vi "ALTS-2015 Prev Test Result Read DB Driver.vi"(7 "Cases":T1, 8 "error in (no error)":errorcluster, 11 "Serial Number":string) -> (0 "error out":errorcluster, 1 "Prev AirLeak result":string, 2 "Non-Empty Data from DB?":bool, 3 "data":string[][](array[string]))   [LabVIEW 2013]
doc: "Copyright © 2005, Soliton Technologies.\nAll rights reserved."
uses:
  <vilib>/addons/database/Auxilliary.llb/DB Tools Parameter Info.ctl
  <vilib>/addons/database/Auxilliary.llb/DB Tools DataTypes.ctl
  <vilib>/addons/database/Auxilliary.llb/DB Tools Parameter Dir.ctl
  Controls/ALTS-2015 Prev Test Result Read DB Driver Options.ctl
  7 Spindle System/Software/Source Code/Controls/7 Spindle - LV2GBL Options.ctl
  <vilib>/addons/database/Command.llb/Cmd ObjectReference.ctl
  <vilib>/addons/database/Connection.llb/DB Tools Open Connec (Path).vi
  <vilib>/addons/database/Command.llb/Cmd Set Parameter Value (C).vi
  <vilib>/addons/database/Command.llb/Cmd Execute.vi
  <vilib>/addons/database/Recordset.llb/Rec Destroy - Connection.vi
  <vilib>/addons/database/Command.llb/Cmd Delete.vi
  <vilib>/addons/database/NI_Database_API.lvlib
panel:
  out "DB Procedure- Data Read":string
  out "parameters out":T2[](array[typedef])
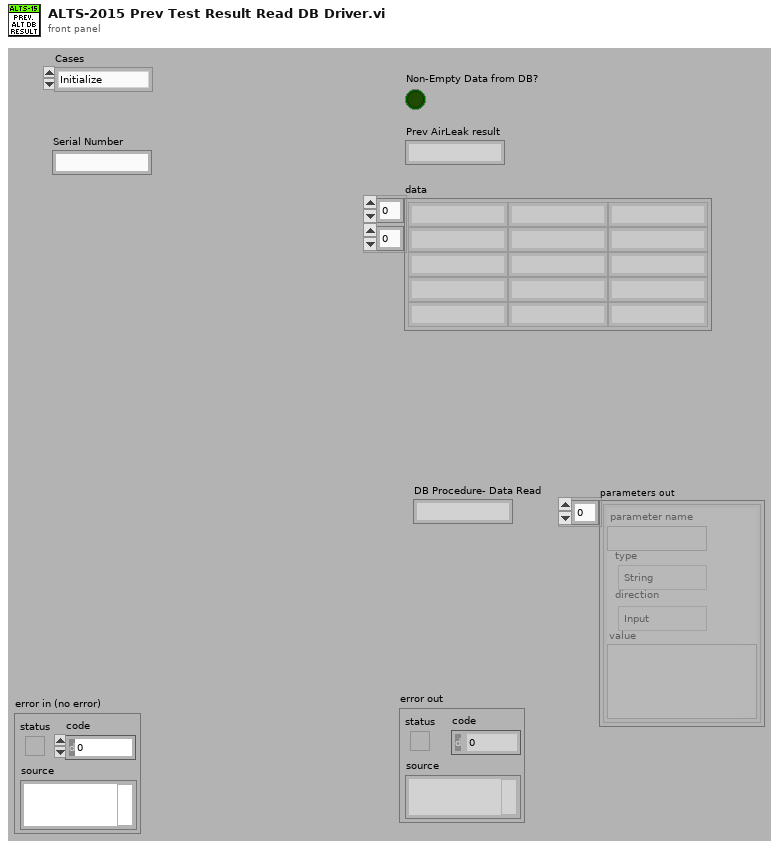
[diagram p1: front panel]
types:
  T1 = typedef "ALTS-2015 Prev Test Result Read DB Driver Options.ctl" = enum16{"Initialize", "Read Table", "Close"}
  T2 = typedef "NI_Database_API.lvlib/DB Tools Parameter Info.ctl" = cluster{"parameter name":string, "type":T3, "direction":T4, "value":variant}
  T3 = typedef "NI_Database_API.lvlib/DB Tools DataTypes.ctl" = enum16{"String", "Long (I32)", "Single (SGL)", "Double (DBL)", "Date/Time", "Binary"}
  T4 = typedef "NI_Database_API.lvlib/DB Tools Parameter Dir.ctl" = enum32{"Input", "Output", "Input/Output", "Return Value"}
  T5 = typedef "7 Spindle - LV2GBL Options.ctl" = enum16{"Read all", "Write all"}
  T6 = typedef "ALTS-2015 INI Configuration Cluster.ctl" = cluster{"Station Details":cluster{"Sensor Name 1":string, "Sensor Name 2":string, "Sensor Name 3":string, "Sensor Name 4":string, "Station1 Enable":bool, "Station2 Enable":bool, "Station3 Enable":bool, "Station4 Enable":bool}, "Database":cluster{"Database Connection Link":path, "Result Procedure":string, "User":string, "Password":string, "Prompt":bool, "Station 1 LT Result DB DSN Path":path, "Station 2 LT Result DB DSN Path":path, "Station 3 LT Result DB DSN Path":path, "Station 4 LT Result DB DSN Path":path, "AirLeakTestResult Procedure":string}, "Simulation":cluster{"Simulate DAQ Hardware":bool, "Simulate Result DB Write":bool, "Scanner Simulation":bool, "Simu. Scanner Path":path, "Simulate OPC":bool, "Simulate LeakTek DB":bool}, "Barcode Scanner1":cluster{"Scanner IP":string, "Scanner Port":u16, "#Bytes to Read":i32}, "Barcode Scanner2":cluster{"Enabled?":bool, "Scanner IP":string, "Scanner Port":u16, "#Bytes to Read":i32}}
  T7 = typedef "NI_Database_API.lvlib/Conn ObjectReference.ctl" = refnum<k1>
  T8 = typedef "NI_Database_API.lvlib/Cmd ObjectReference.ctl" = refnum<k1>
  T9 = typedef "NI_Database_API.lvlib/Cmd-Rec Object Reference.ctl" = refnum<k1>
  T10 = typedef "NI_Database_API.lvlib/Cmd-Rec Data Members.ctl" = cluster{"recordset reference":T11, "command reference":T8}
  T11 = typedef "NI_Database_API.lvlib/Rec ObjectReference.ctl" = refnum<k1>
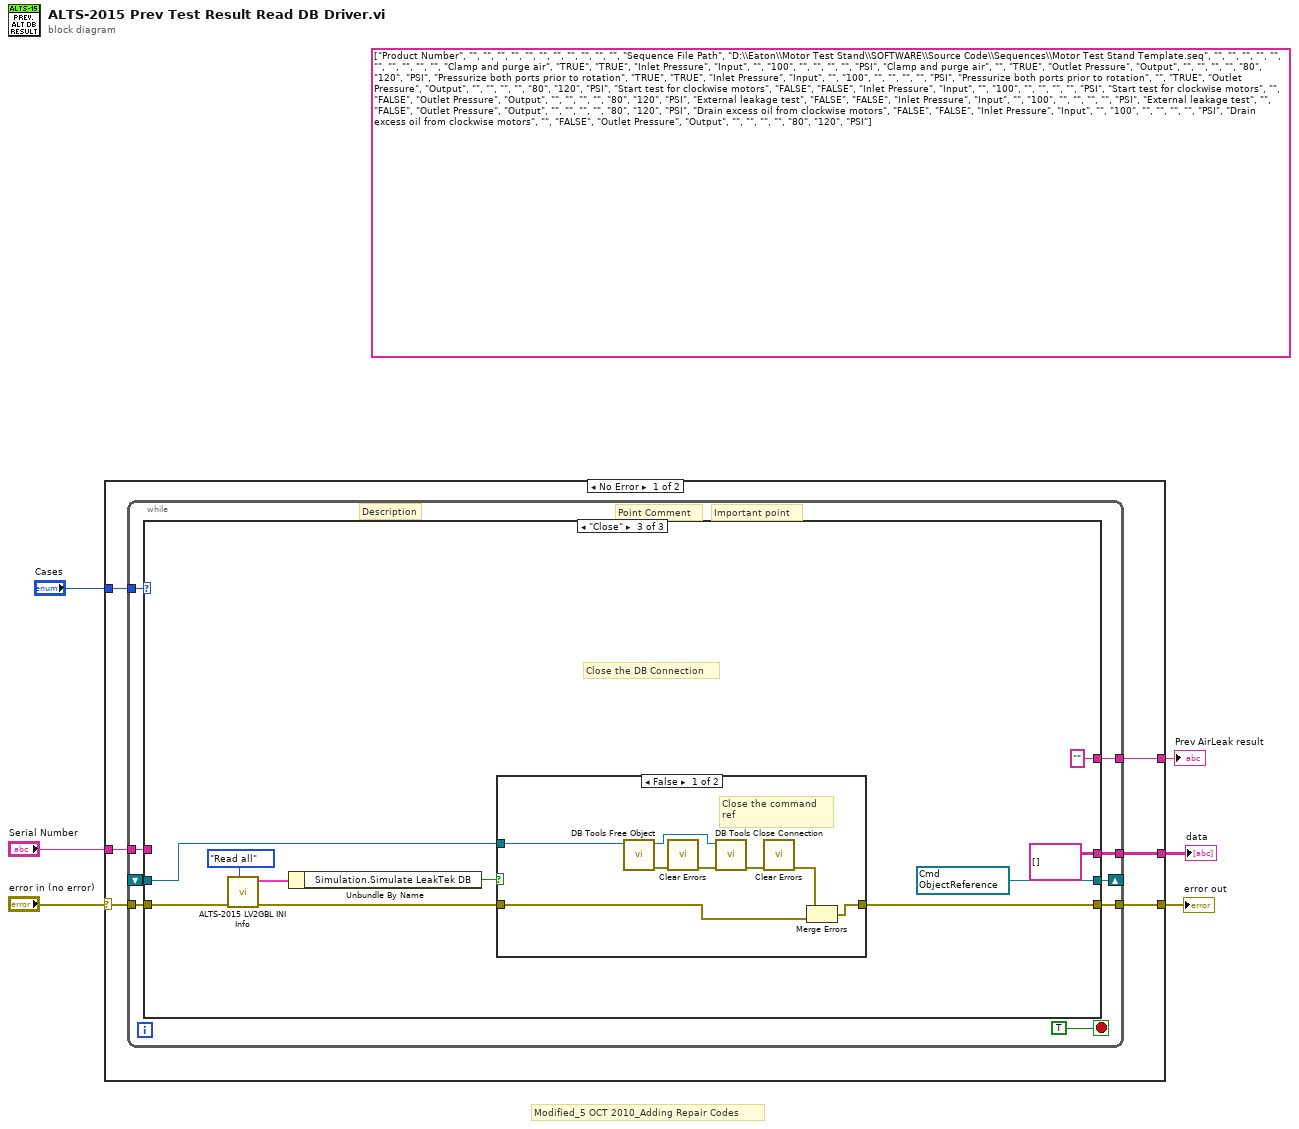
[diagram p0: block diagram]
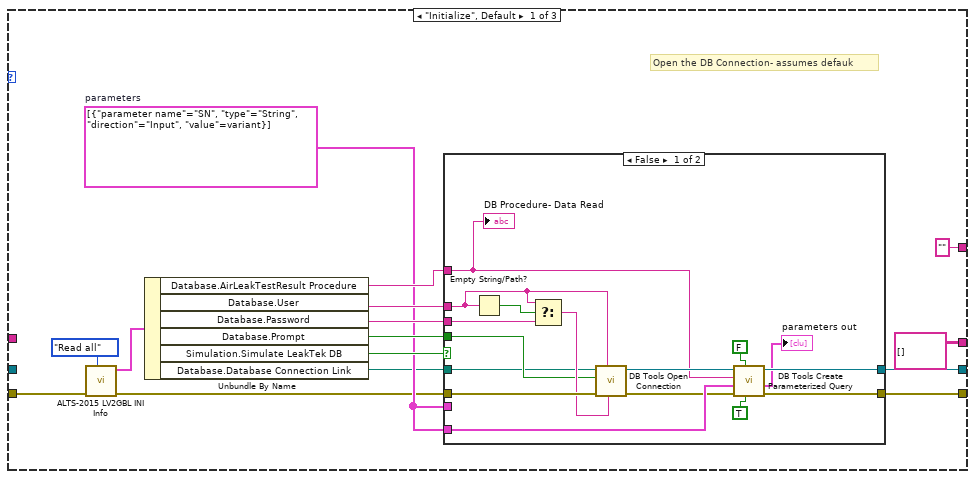
[diagram p2: hidden frame]
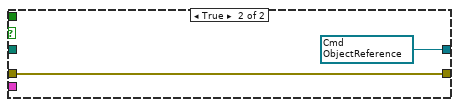
[diagram p3: hidden frame]
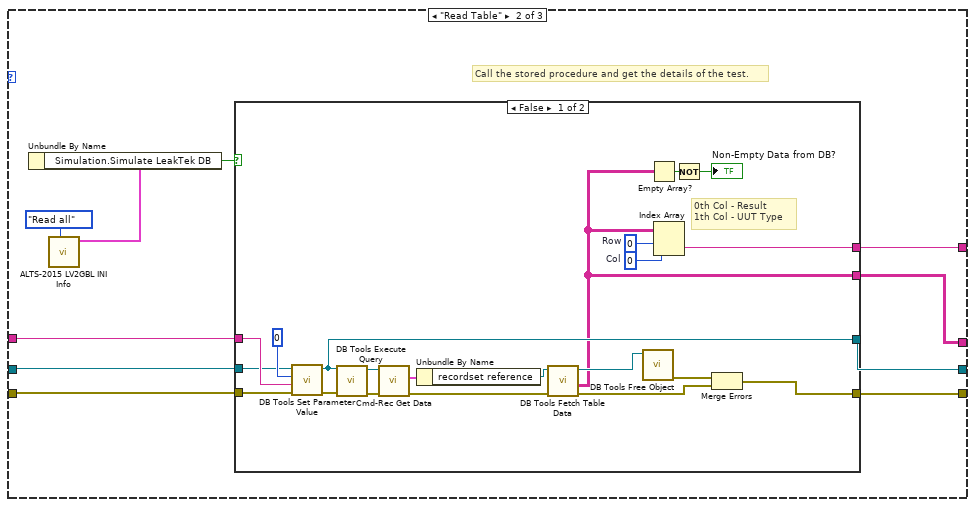
[diagram p4: hidden frame]
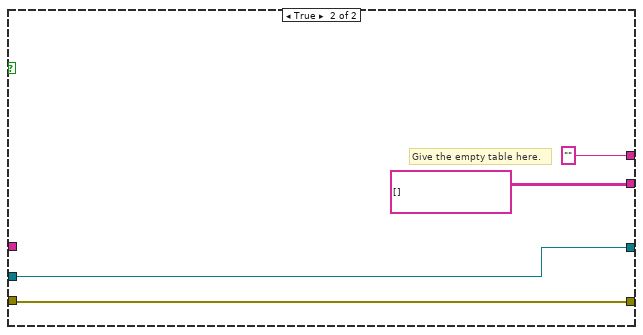
[diagram p5: hidden frame]
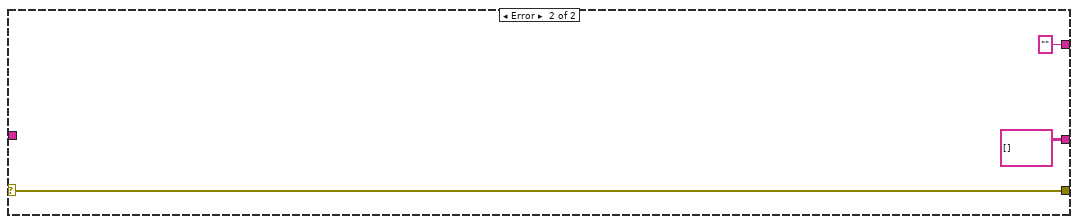
[diagram p7: hidden frame]
diagram:
  (unwired) string[][] [["Product Number", "", "", "", "", "", "", "", "", "", "", ""], ["Sequence File Path", "D:\\Eaton\\Motor Test Stand\\SOFTWARE\\Source Code\\Sequences\\Motor Test Stand Template.seq", "", "", "", "", "", "", "", "", "", ""], ["Clamp and purge air", "TRUE", "TRUE", "Inlet Pressure", "Input", "", "100", "", "", "", "", "PSI"], ["Clamp and purge air", "", "TRUE", "Outlet Pressure", "Output", "", "", "", "", "80", "120", "PSI"], ["Pressurize both ports prior to rotation", "TRUE", "TRUE", "Inlet Pressure", "Input", "", "100", "", "", "", "", "PSI"], ["Pressurize both ports prior to rotation", "", "TRUE", "Outlet Pressure", "Output", "", "", "", "", "80", "120", "PSI"], ["Start test for clockwise motors", "FALSE", "FALSE", "Inlet Pressure", "Input", "", "100", "", "", "", "", "PSI"], ["Start test for clockwise motors", "", "FALSE", "Outlet Pressure", "Output", "", "", "", "", "80", "120", "PSI"], ["External leakage test", "FALSE", "FALSE", "Inlet Pressure", "Input", "", "100", "", "", "", "", "PSI"], ["External leakage test", "", "FALSE", "Outlet Pressure", "Output", "", "", "", "", "80", "120", "PSI"], ["Drain excess oil from clockwise motors", "FALSE", "FALSE", "Inlet Pressure", "Input", "", "100", "", "", "", "", "PSI"], ["Drain excess oil from clockwise motors", "", "FALSE", "Outlet Pressure", "Output", "", "", "", "", "80", "120", "PSI"]] ("appended array")
  # "Modified_5 OCT 2010_Adding Repair Codes"
  n1 = case shown="No Error" "error in (no error)" {
    selector: "error in (no error)" -> [w11 w111]
    tunnel: [w12 w111] -> w5
    tunnel: "Cases" -> [w10 _]
    tunnel: [w9 string[][] []] -> w4
    tunnel: "Serial Number" -> [w8 _]
    tunnel: [w7 "" ("String")] -> w1
    frame No Error {
      # "Point Comment"
      # "Important point"
      # "Description"
      n2 = while {
        tunnel: [w20] -> w12
        shift-right: [w19] -> _
        shift-left: _ -> [w18]
        tunnel: w11 -> [w17]
        tunnel: w10 -> [w16]
        tunnel: [w15] -> w9
        tunnel: w8 -> [w14]
        tunnel: [w13] -> w7
        stop <- TRUE stop-if-true
        n3 = case shown="\"Close\"" w16 {
          tunnel: w17 -> [w25 w63 w93]
          tunnel: [w36 w64 w99] -> w20
          tunnel: [w35 w58 w96] -> w19
          tunnel: w18 -> [_ w59 w97]
          tunnel: [string[][] [] w60 string[][] []] -> w15
          tunnel: w14 -> [_ w61 _]
          tunnel: ["" ("String") w57 "" ("String")] -> w13
          frame "Initialize", Default {
            w28 = T2[] [{"parameter name"="SN", "type"=enum."String", "direction"=enum."Input", "value"=variant}]  # parameters
            # "Open the DB Connection- assumes defauk"
            n4 = call "ALTS-2015 LV2GBL INI Info.vi"("Options"=7_Spindle_-_LV2GBL_Options."Read all", "error in"=w25) -> ("error out"=w24:errorcluster, "Configuration Cluster Out"=w23:T6)  [unwired: 8 in]
            n5 = Unbundle By Name(w23) -> ("Database.AirLeakTestResult Procedure"=w29:string, "Database.User"=w32:string, "Database.Password"=w31:string, "Database.Prompt"=w30:bool, "Simulation.Simulate LeakTek DB"=w33:bool, "Database.Database Connection Link"=w27:path)
            n6 = case shown="False" w33 {
              tunnel: [w40 w54] -> w36
              tunnel: [w43 w53] -> w35
              tunnel: w27 -> [w37 _]
              tunnel: w24 -> [w52 w54]
              tunnel: w32 -> [w49 _]
              tunnel: w31 -> [w48 _]
              tunnel: w30 -> [w47 _]
              tunnel: w29 -> [w39 _]
              tunnel: w28 -> [w42 _]
              tunnel: w28 -> [_ _]
              frame False {
                n7 = Empty String/Path?(string/path=w49) -> (empty?=w51:bool)
                n8 = Select(t=w49, s=w51, f=w48) -> (s? t:f=w50:string)
                n9 = call-poly <vilib>:"DB Tools Open Connection.vi"("password"=w50, "userID"=w49, "error in (no error)"=w52, "prompt? (F)"=w47, "connection information"=w37) -> ("error out"=w41:errorcluster, "connection reference"=w44:T7)  [unwired: 3 in]
                n10 = call <vilib>:"DB Tools Create Parameterized Query.vi"("stored procedure? (F)"=TRUE ("stored procedure? (f)"), "auto-detect parameters? (F)"=FALSE ("auto-detect parameters? (f)"), "error in (no error)"=w41, "parameters"=w42, "SQL query"=w39, "connection reference"=w44) -> ("error out"=w40:errorcluster, "parameters out"=→"parameters out":T2[], "command reference"=w43:T8)  [unwired: 1 in]
                "DB Procedure- Data Read" <- w39
              }
              frame True {
                w53 = T8 refnum items=["Command"] ("command reference")
              }
            }
          }
          frame "Read Table" {
            # "Call the stored procedure and get the details of the test."
            n11 = call "ALTS-2015 LV2GBL INI Info.vi"("Options"=7_Spindle_-_LV2GBL_Options."Read all") -> ("Configuration Cluster Out"=w56:T6)  [unwired: 9 in, 1 out]
            n12 = Unbundle By Name(w56) -> ("Simulation.Simulate LeakTek DB"=w62:bool)
            n13 = case shown="False" w62 {
              tunnel: [w80 w89] -> w64
              tunnel: [w68 string[][] [] ("recordset data")] -> w60
              tunnel: w63 -> [w78 w89]
              tunnel: w59 -> [w77 w88]
              tunnel: w61 -> [w84 _]
              tunnel: [w69 w88] -> w58
              tunnel: [w65 "" ("String")] -> w57
              frame False {
                w66 = 0  # Col
                w67 = 0  # Row
                # "0th Col - Result\n1th Col - UUT Type"
                n14 = call-poly <vilib>:"DB Tools Set Parameter Value.vi"("error in (no error)"=w78, "value"=w84, "parameter index"=0, "command reference"=w77) -> ("error out"=w81:errorcluster, "command reference out"=w69:T8)  [unwired: 4 in]
                n15 = call-poly <vilib>:"DB Tools Execute Query.vi"("error in (no error)"=w81, "command reference"=w69) -> ("error out"=w75:errorcluster, "command-recordset reference"=w70:T9)  [unwired: 6 in]
                n16 = call <vilib>:"Cmd-Rec Get Data.vi"("error in (no error)"=w75, "command-recordset reference"=w70) -> ("error out"=w71:errorcluster, "data"=w76:T10)  [unwired: 2 in, 2 out]
                n17 = Unbundle By Name(w76) -> ("recordset reference"=w74:T11)
                n18 = call <vilib>:"DB Tools Fetch Table Data.vi"("error in (no error)"=w71, "recordset reference"=w74) -> ("error out"=w72:errorcluster, "recordset data"=w68:string[][], "recordset reference out"=w73:T11)  [unwired: 3 in]
                n19 = call-poly <vilib>:"DB Tools Free Object.vi"("recordset reference"=w73) -> ("error out"=w79:errorcluster)  [unwired: 9 in, 1 out]
                n20 = Empty Array?(array=w68) -> (empty?=w83:bool)
                n21 = Index Array(array=w68, index (row)=w67, index (col)=w66) -> (element=w65:string)
                n22 = Not(x=w83) -> (.not. x?=→"Non-Empty Data from DB?":bool)
                n23 = Merge Errors(w79, w72) -> (w80:errorcluster)
              }
              frame True {
                # "Give the empty table here."
              }
            }
          }
          frame "Close" {
            w96 = T8 refnum items=["Command"] ("command reference")
            # "Close the DB Connection"
            n24 = call "ALTS-2015 LV2GBL INI Info.vi"("Options"=7_Spindle_-_LV2GBL_Options."Read all", "error in"=w93) -> ("error out"=w92:errorcluster, "Configuration Cluster Out"=w91:T6)  [unwired: 8 in]
            n25 = Unbundle By Name(w91) -> ("Simulation.Simulate LeakTek DB"=w95:bool)
            n26 = case shown="False" w95 {
              tunnel: [w105 w108] -> w99
              tunnel: w92 -> [w106 w108]
              tunnel: w97 -> [w103 _]
              frame False {
                # "Close the command ref"
                n27 = call-poly <vilib>:"DB Tools Free Object.vi"("command reference"=w103) -> ("error out"=w102:errorcluster, "connection reference"=w100:T7)  [unwired: 9 in]
                n28 = call <vilib>:"Clear Errors.vi"("error in (no error)"=w102) -> ("error out"=w101:errorcluster)  [unwired: 6 in]
                n29 = call <vilib>:"DB Tools Close Connection.vi"("error in (no error)"=w101, "connection reference"=w100) -> ("error out"=w107:errorcluster)  [unwired: 5 in]
                n30 = call <vilib>:"Clear Errors.vi"("error in (no error)"=w107) -> ("error out"=w104:errorcluster)  [unwired: 6 in]
                n31 = Merge Errors(w104, w106) -> (w105:errorcluster)
              }
              frame True {
              }
            }
          }
        }
      }
    }
    frame Error {
    }
  }
  "error out" <- w5
  "data" <- w4
  "Prev AirLeak result" <- w1
